vi "ExADCGbl.vi"() -> ()   [LabVIEW 2010]
uses:
  Open-Close Hardware/CamHandle.vi
panel:
  out "Pixel Time":i32
  out "Bit Depth":i32
  out "ReadOut port":i32
  out "ADC Offset":i32
  out "ADC Gain":i32
  out "ADC Speed":i32
  in  "Readout Port":i32=2 min=-1 step=1
  in  "ADC Offset":i32=-1 min=-1 step=1
  in  "ADC Gain":i32=2 min=-1 step=1
  in  "ADC speed":i32=-2 min=-3 step=1
  out "error out":errorcluster
  in  "error in (no error)":errorcluster
  # "ExADCGbl:\nThis program shows how to use the  CameraADCset.vi and the CameraADCget.vi. This example allows all the ADC settings to be set or ignored."
  # "The following are read \nfrom camera after setting\nvalues to left.\n-1 value means it isn't \nsupported by camera."
  # "For Slowest ADC speed set this to -3\nFor Fastest ADC speed set this to -2\nTo use current ADC speed don't  hook up or use -1\notherwise put speed in as kHz"
  # "To use current gain don't hook up or set to -1"
  # "To use current gain don't hook up or set to -1"
  # "To use current gain don't hook up or set to -1"
  # "NOTICE\n\nTHIS VI USES A GLOBAL CAMERA HANDLE\n\nTHE VI EXOPENGLOBALCAM.VI MUST BE\nRUN AT THE START OF THE WORK SESSION.\nTHE CAMERA WILL REMAIN OPENED.\n\nTHE VI EXCLOSEGLOBALCAM.VI MUST\nBE RUN BEFORE LEAVING LABVIEW."
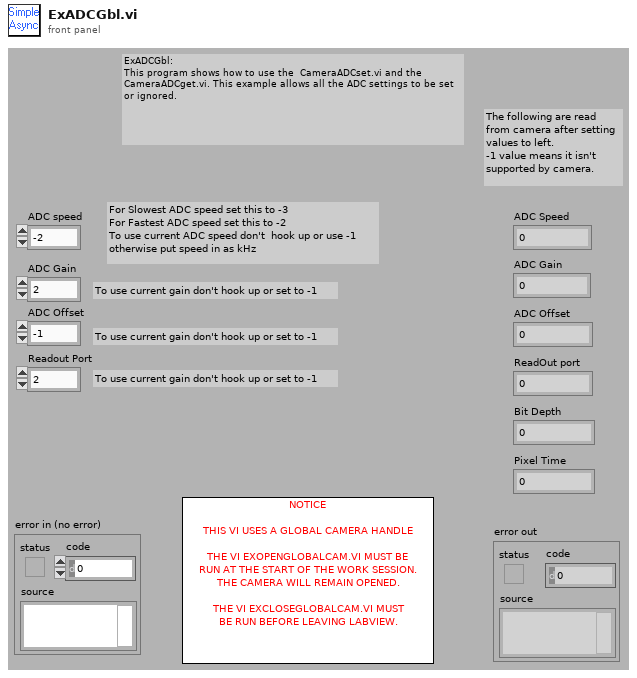
[diagram p1: front panel]
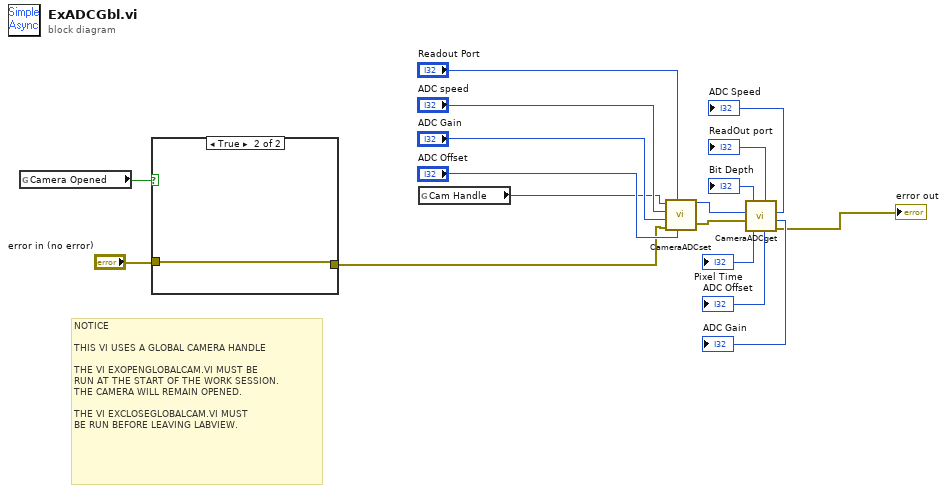
[diagram p0: block diagram]
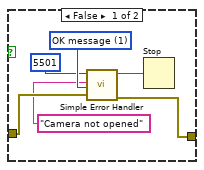
[diagram p2: hidden frame]
diagram:
  # "NOTICE\n\nTHIS VI USES A GLOBAL CAMERA HANDLE\n\nTHE VI EXOPENGLOBALCAM.VI MUST BE\nRUN AT THE START OF THE WORK SESSION.\nTHE CAMERA WILL REMAIN OPENED.\n\nTHE VI EXCLOSEGLOBALCAM.VI MUST\nBE RUN BEFORE LEAVING LABVIEW."
  n1 = global read "CamHandle.vi" "Camera Opened"() -> (w5:bool)
  n2 = case shown="True" w5 {
    tunnel: "error in (no error)" -> [w22 w24]
    tunnel: [w21 w24] -> w2
    frame False {
      w23 = u16 1 items=["no dialog", "OK message", "continue or stop message"] ("type of dialog (OK msg:1)")
      n3 = call <vilib>:"Simple Error Handler.vi"("error code (no error:0)"=5501, "error source (\" \")"="Camera not opened", "type of dialog (OK msg:1)"=w23, "error in (no error)"=w22) -> ("error?"=w19:bool, "error out"=w21:errorcluster)  [unwired: 1 in, 3 out]
      n4 = Stop(stop? (T)=w19) -> ()
    }
    frame True {
    }
  }
  n5 = global read "CamHandle.vi" "Cam Handle"() -> (w3:u32)
  n6 = call <userlib>:"CameraADCset.vi"("ADC offset"="ADC Offset", "Read Out port"="Readout Port", "error in (no error)"=w2, "ADC Gain"="ADC Gain", "ADC Speed"="ADC speed", "Camera Handle"=w3) -> ("error out"=w11:errorcluster, "Camera Handle"=w12:u32)
  n7 = call <userlib>:"CameraADCget.vi"("Camera handle"=w12, "error in (no error)"=w11) -> ("Bit Depth"=→"Bit Depth":i32, "Pixel Time"=→"Pixel Time":i32, "Readout Port"=→"ReadOut port":i32, "ADC Offset"=→"ADC Offset":i32, "ADC Speed"=→"ADC Speed":i32, "ADC Gain"=→"ADC Gain":i32, "error out"=→"error out":errorcluster)  [unwired: 1 out]
